vi "Read&Write ini.vi"(0 "功能":enum16{"读取配置", "写入配置"}(ring), 5 "configuration file path":path caption="配置文件的路径", 7 "section":string caption="段", 9 "key":string caption="键", 11 "key 2":string caption="值:In") -> (4 "key 4":string caption="值：Out")   [LabVIEW 2013]
uses:
  <vilib>/Utility/config.llb/Write Key (String).vi
  <vilib>/Utility/config.llb/Read Key (String).vi
  <vilib>/Utility/config.llb/NI_LVConfig.lvlib
panel:
  out "error out":errorcluster caption="错误输出"
  in  "error in (no error)":errorcluster caption="错误输入（无错误）"
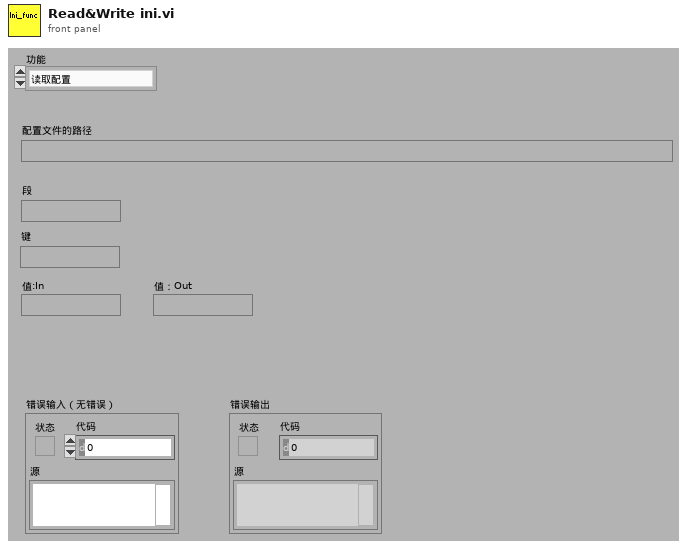
[diagram p1: front panel]
types:
  T1 = typedef "NI_LVConfig.lvlib/Config Data RefNum.ctl" = refnum<k1>
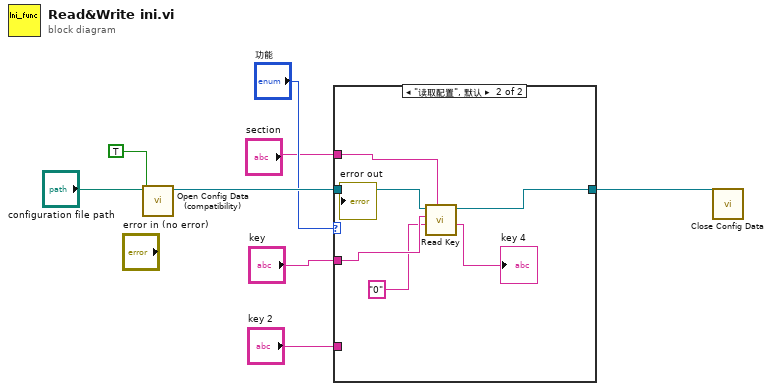
[diagram p0: block diagram]
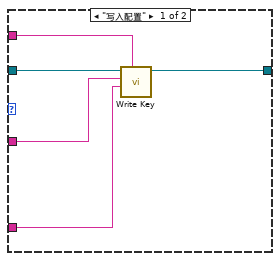
[diagram p2: hidden frame]
diagram:
  n1 = call <vilib>:"Open Config Data (compatibility).vi"("create file if necessary (T)"=TRUE ("create file if necessary? (T)"), "configuration file path"="configuration file path") -> ("refnum"=w8:T1)  [unwired: 7 in, 2 out]
  n2 = case shown="\"读取配置\", 默认" "功能" {
    tunnel: w8 -> [w13 w19]
    tunnel: [w12 w14] -> w4
    tunnel: "section" -> [w11 w18]
    tunnel: "key" -> [w10 w16]
    tunnel: "key 2" -> [w9 _]
    frame "写入配置" {
      n3 = call-poly <vilib>:"Write Key.vi"("section"=w11, "value"=w9, "key"=w10, "refnum"=w13) -> ("refnum out"=w12:T1)  [unwired: 2 in, 5 out]
    }
    frame "读取配置", Default {
      n4 = call-poly <vilib>:"Read Key.vi"("section"=w18, "default value"="0", "key"=w16, "refnum"=w19) -> ("value"=→"key 4":string, "refnum out"=w14:T1)  [unwired: 2 in, 4 out]
    }
  }
  n5 = call <vilib>:"Close Config Data.vi"("refnum"=w4) -> ()  [unwired: 2 in, 9 out]
